vi "configuration class to cluster.vi"(8 "error in (no error)":errorcluster, 11 "DSFConfiguration in":refnum<class "DSFConfiguration.lvclass">) -> (0 "error out":errorcluster, 3 "configuration cluster":T5)   [LabVIEW 2017, in "DSFConfiguration.lvclass"]
uses:
  DSFConfiguration.lvclass
  Controls/dsf timing.ctl
  Controls/dsf transfer.ctl
  Controls/dsf channel.ctl
  Controls/dsf settings.ctl
  DSFConfiguration.lvclass/DSFConfiguration.ctl
  IDable/IDable.lvclass/IDable.ctl
  DSFPlugin/DSFPlugin.lvclass/DSFPlugin.ctl
  DSFPluginSettings/DSFPluginSettings.lvclass/DSFPluginSettings.ctl
  DSFChannel/DSFChannel.lvclass/DSFChannel.ctl
  DSFTransfer/DSFTransfer.lvclass/DSFTransfer.ctl
  DSFGroup/DSFGroup.lvclass/DSFGroup.ctl
  IDable/Read id.vi
  DSFPluginSettings/Read plugin settings info.vi
  DSFChannel/Read channel info.vi
  DSFTransfer/Read transfer info.vi
  DSFGroup/Read group info.vi
  DSFPlugin/Read plugin info.vi
  Read plugins.vi
  Read groups.vi
  Read transfers.vi
  Read channels.vi
  Read settings.vi
  DSFPluginSettings/DSFPluginSettings.lvclass
  C:/github/data-sharing-framework/Source/Configuration API/Classes/IDable/IDable.lvclass
  DSFChannel/DSFChannel.lvclass
  DSFTransfer/DSFTransfer.lvclass
  DSFGroup/DSFGroup.lvclass
  DSFPlugin/DSFPlugin.lvclass
  DSFTiming/Get Timing Information.vi
  DSFTiming/DSFTiming.lvclass
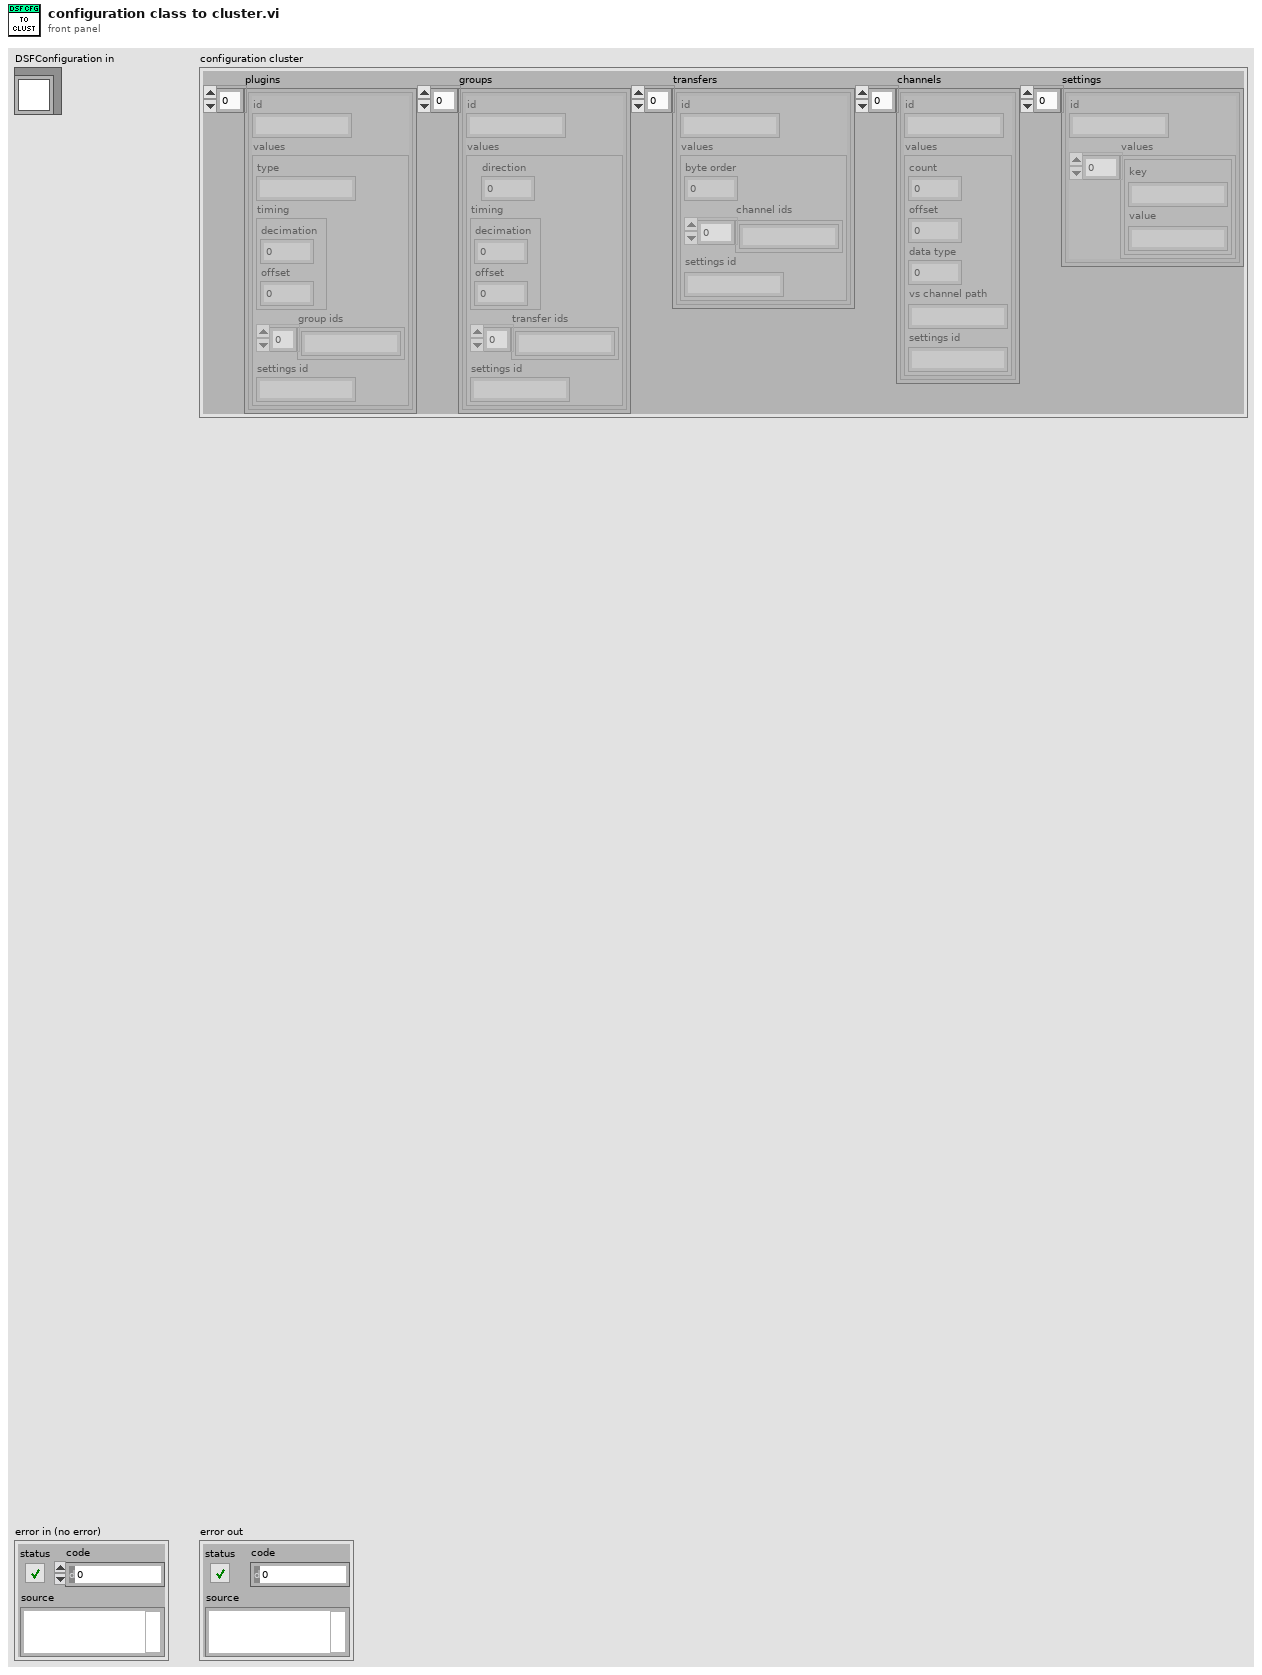
[diagram p1: front panel]
types:
  T1 = typedef "dsf timing.ctl" = cluster{"decimation":i32, "offset":i32}
  T2 = typedef "dsf transfer.ctl" = cluster{"byte order":i32, "channel ids":string[], "settings id":string}
  T3 = typedef "dsf channel.ctl" = cluster{"count":i32, "offset":i32, "data type":i32, "vs channel path":string, "settings id":string}
  T4 = typedef "dsf settings.ctl" = cluster{"key":string, "value":string}[]
  T5 = cluster{"plugins":cluster{"id":string, "values":cluster{"type":string, "timing":T1, "group ids":string[], "settings id":string}}[], "groups":cluster{"id":string, "values":cluster{"direction":i32, "timing":T1, "transfer ids":string[], "settings id":string}}[], "transfers":cluster{"id":string, "values":T2}[], "channels":cluster{"id":string, "values":T3}[], "settings":cluster{"id":string, "values":T4}[]}
  T6 = cluster{"direction":string, "timing":T1, "transfer ids":string[], "settings id":string}
  T7 = typedef "dsf plugin.ctl" = cluster{"type":string, "timing":refnum<class "DSFTiming.lvclass">, "groups ids":string[], "settings id":string}
  T8 = cluster{"accessors:id":string, "group info":cluster{"direction":string, "timing":T1, "transfer ids":string[], "settings id":string}}
  T9 = cluster{"direction":i32, "timing":T1, "transfer ids":string[], "settings id":string}
  T10 = typedef "dsf group.ctl" = cluster{"direction":i32, "timing":refnum<class "DSFTiming.lvclass">, "transfer ids":string[], "settings id":string}
  T11 = cluster{"accessors:id":string, "group info":cluster{"direction":i32, "timing":T1, "transfer ids":string[], "settings id":string}}
  T12 = cluster{"accessors:id":string, "accessors:transfer info":T2}
  T13 = cluster{"accessors:id":string, "accessors:channel info":T3}
  T14 = cluster{"accessors:id":string, "accessors:plugin settings info":T4}
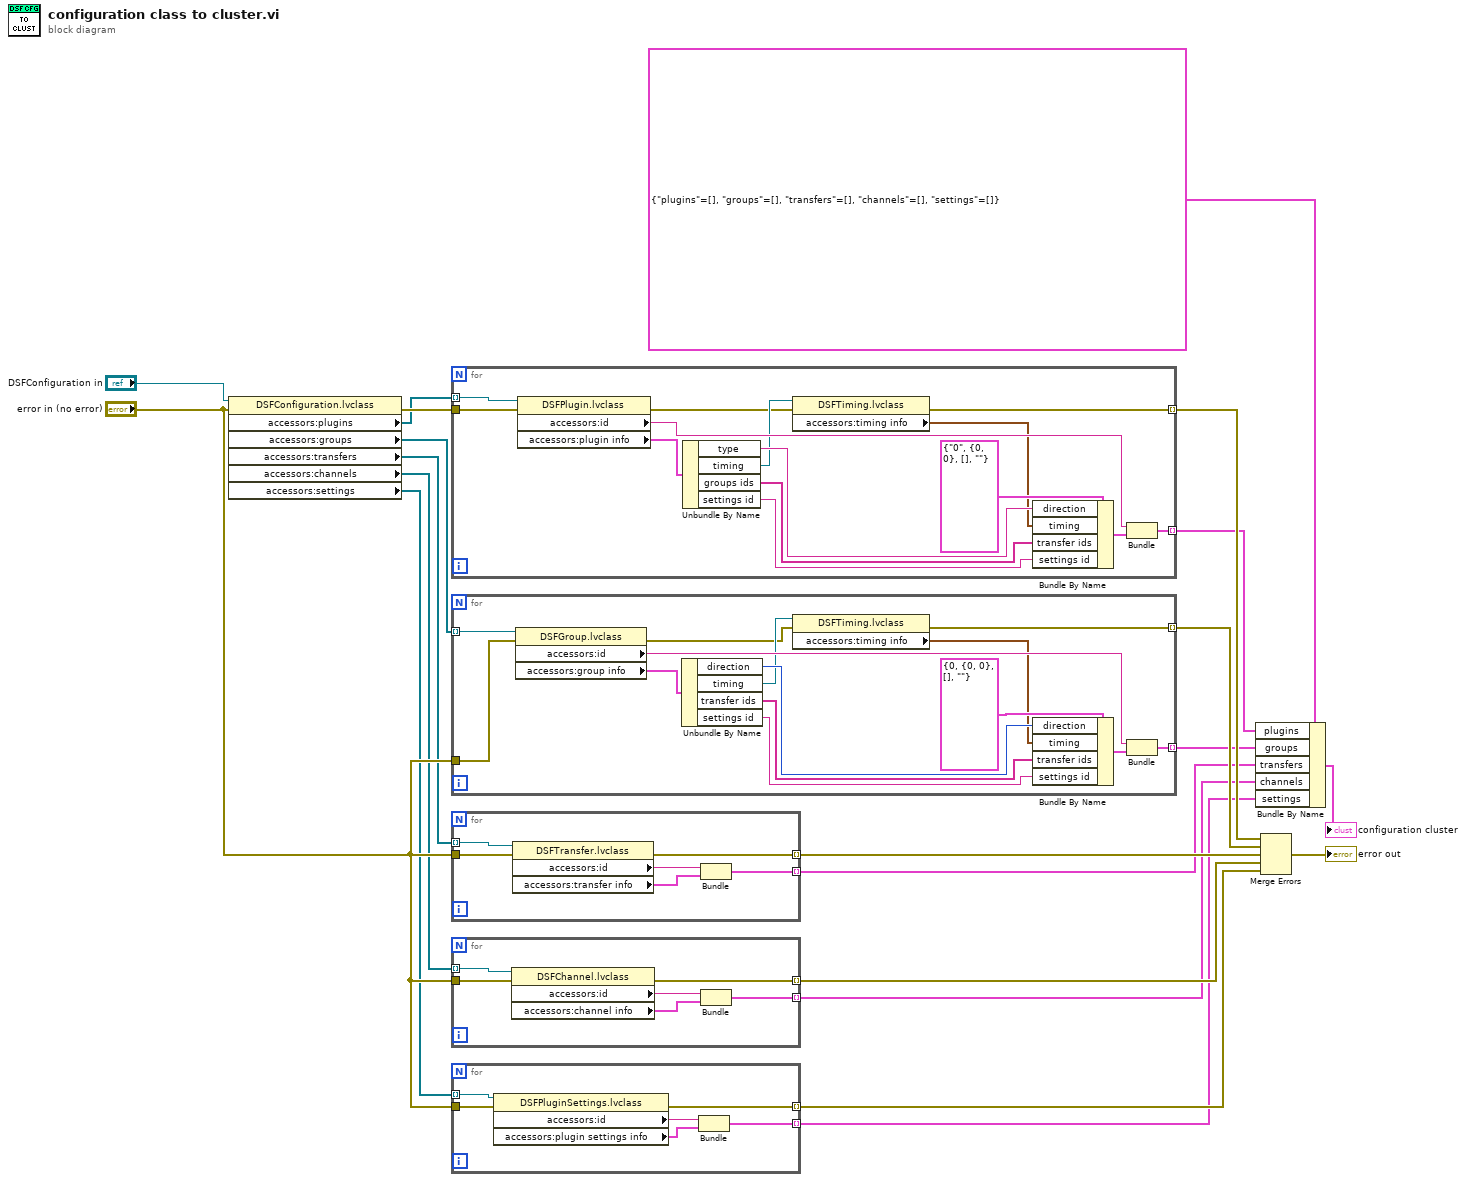
[diagram p0: block diagram]
diagram:
  n1 = property class="DSFConfiguration.lvclass"(reference="DSFConfiguration in", error in="error in (no error)") -> (error out=w14:errorcluster, "accessors:plugins"=w12:refnum<class "DSFPlugin.lvclass">[], "accessors:groups"=w10:refnum<class "DSFGroup.lvclass">[], "accessors:transfers"=w8:refnum<class "DSFTransfer.lvclass">[], "accessors:channels"=w6:refnum<class "DSFChannel.lvclass">[], "accessors:settings"=w7:refnum<class "DSFPluginSettings.lvclass">[])  [unwired: 1 out]
  n2 = for {
    tunnel: w12 -> [w35] mode=indexing
    tunnel: [w33] -> w13 mode=indexing
    tunnel: w14 -> [w24]
    tunnel: [w22] -> w15 mode=indexing
    n3 = property class="DSFPlugin.lvclass"(reference=w35, error in=w24) -> (error out=w23:errorcluster, "accessors:id"=w34:string, "accessors:plugin info"=w32:T7)  [unwired: 1 out]
    n4 = Unbundle By Name(w32) -> ("type"=w29:string, "timing"=w28:refnum<class "DSFTiming.lvclass">, "groups ids"=w26:string[], "settings id"=w25:string)
    n5 = property class="DSFTiming.lvclass"(reference=w28, error in=w23) -> (error out=w22:errorcluster, "accessors:timing info"=w27:T1)  [unwired: 1 out]
    n6 = Bundle By Name(cluster=T6 {"direction"="0", "timing"={"decimation"=0, "offset"=0}, "transfer ids"=[], "settings id"=""} ("group info"), "direction"=w29, "timing"=w27, "transfer ids"=w26, "settings id"=w25) -> (w30:T6)
    n7 = Bundle("accessors:id"=w34, "group info"=w30) -> (w33:T8)  [unwired: 1 in]
  }
  n8 = for {
    tunnel: w10 -> [w49] mode=indexing
    tunnel: [w47] -> w11 mode=indexing
    tunnel: "error in (no error)" -> [w38]
    tunnel: [w36] -> w16 mode=indexing
    n9 = property class="DSFGroup.lvclass"(reference=w49, error in=w38) -> (error out=w37:errorcluster, "accessors:id"=w48:string, "accessors:group info"=w46:T10)  [unwired: 1 out]
    n10 = Unbundle By Name(w46) -> ("direction"=w43:i32, "timing"=w42:refnum<class "DSFTiming.lvclass">, "transfer ids"=w40:string[], "settings id"=w39:string)
    n11 = property class="DSFTiming.lvclass"(reference=w42, error in=w37) -> (error out=w36:errorcluster, "accessors:timing info"=w41:T1)  [unwired: 1 out]
    n12 = Bundle By Name(cluster=T9 {"direction"=0, "timing"={"decimation"=0, "offset"=0}, "transfer ids"=[], "settings id"=""} ("group info"), "direction"=w43, "timing"=w41, "transfer ids"=w40, "settings id"=w39) -> (w44:T9)
    n13 = Bundle("accessors:id"=w48, "group info"=w44) -> (w47:T11)  [unwired: 1 in]
  }
  n14 = for {
    tunnel: w8 -> [w55] mode=indexing
    tunnel: [w52] -> w9 mode=indexing
    tunnel: "error in (no error)" -> [w51]
    tunnel: [w50] -> w17 mode=indexing
    n15 = property class="DSFTransfer.lvclass"(reference=w55, error in=w51) -> (error out=w50:errorcluster, "accessors:id"=w54:string, "accessors:transfer info"=w53:T2)  [unwired: 1 out]
    n16 = Bundle("accessors:id"=w54, "accessors:transfer info"=w53) -> (w52:T12)  [unwired: 1 in]
  }
  n17 = for {
    tunnel: w6 -> [w61] mode=indexing
    tunnel: [w58] -> w4 mode=indexing
    tunnel: "error in (no error)" -> [w57]
    tunnel: [w56] -> w18 mode=indexing
    n18 = property class="DSFChannel.lvclass"(reference=w61, error in=w57) -> (error out=w56:errorcluster, "accessors:id"=w60:string, "accessors:channel info"=w59:T3)  [unwired: 1 out]
    n19 = Bundle("accessors:id"=w60, "accessors:channel info"=w59) -> (w58:T13)  [unwired: 1 in]
  }
  n20 = for {
    tunnel: [w66] -> w5 mode=indexing
    tunnel: w7 -> [w65] mode=indexing
    tunnel: "error in (no error)" -> [w63]
    tunnel: [w62] -> w20 mode=indexing
    n21 = property class="DSFPluginSettings.lvclass"(reference=w65, error in=w63) -> (error out=w62:errorcluster, "accessors:id"=w67:string, "accessors:plugin settings info"=w64:T4)  [unwired: 1 out]
    n22 = Bundle("accessors:id"=w67, "accessors:plugin settings info"=w64) -> (w66:T14)  [unwired: 1 in]
  }
  n23 = Bundle By Name(cluster=T5 {"plugins"=[], "groups"=[], "transfers"=[], "channels"=[], "settings"=[]}, "plugins"=w13, "groups"=w11, "transfers"=w9, "channels"=w4, "settings"=w5) -> (→"configuration cluster":T5)
  n24 = Merge Errors(w15, w16, w17, w18, w20) -> (→"error out":errorcluster)
